vi "get_config_path.vi"(6 "configuration":T1, 8 "error in (no error)":errorcluster, 11 "custom_path":path) -> (0 "error out":errorcluster, 3 "lv_build_config_path":path)   [LabVIEW 2015, in "lv-builder-default.lvlib"]
uses:
  lv-builder-default.lvlib
  public/_controls/configuration.ctl
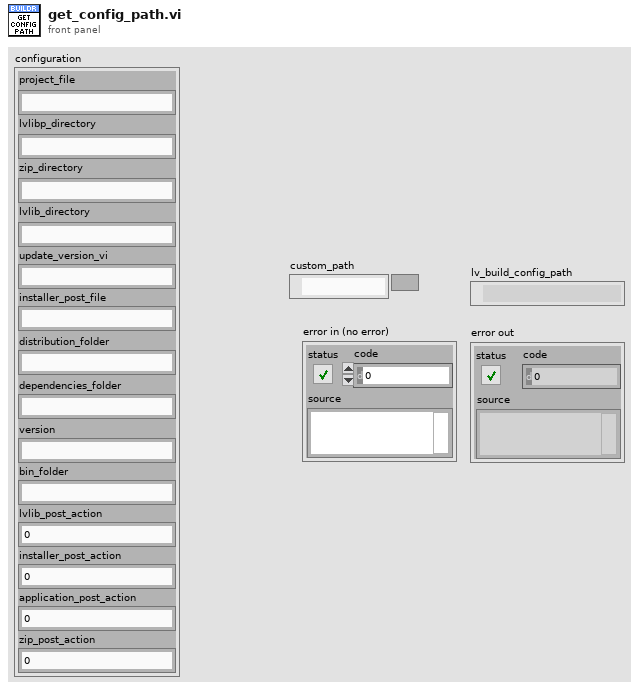
[diagram p1: front panel]
types:
  T1 = typedef "lv-builder-default.lvlib/configuration.ctl" = cluster{"project_file":string, "lvlibp_directory":string, "zip_directory":string, "lvlib_directory":string, "update_version_vi":string, "installer_post_file":string, "distribution_folder":string, "dependencies_folder":string, "version":string, "bin_folder":string, "lvlib_post_action":u16, "installer_post_action":u16, "application_post_action":u16, "zip_post_action":u16}
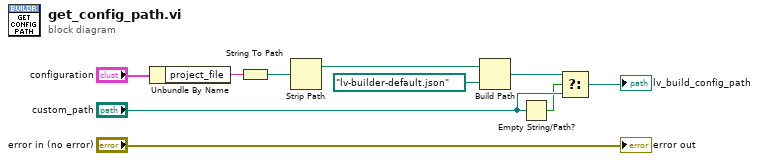
[diagram p0: block diagram]
diagram:
  n1 = Unbundle By Name("configuration") -> ("project_file"=w4:string)
  n2 = String To Path(string=w4) -> (path=w3:path)
  n3 = Strip Path(path=w3) -> (stripped path=w2:path)  [unwired: 1 out]
  n4 = Build Path(base path=w2, name or relative path=path "lv-builder-default.json" ("system directory")) -> (appended path=w9:path)
  n5 = Empty String/Path?(string/path="custom_path") -> (empty?=w6:bool)
  n6 = Select(t=w9, s=w6, f="custom_path") -> (s? t:f=→"lv_build_config_path":path)
  "error out" <- "error in (no error)"
